vi "RealFlight Controller Layout.vi"(2 "JoyStick Name":string) -> (0 "IDLE up":bool, 1 "Left Lower":bool, 3 "IDLE down":bool, 4 "Down":bool, 5 "Gain":dbl(knob) scale=-1.0..1.0, 6 "Right Stick X":dbl, 7 "Right Stick Y":dbl, 8 "Right":bool, 9 "Left Stick Y":dbl, 10 "Left Stick X":dbl)   [LabVIEW 2012]
uses:
  <vilib>/Rock Robotics/WPI/Joystick/WPI_JoystickGetSetRefNum.vi
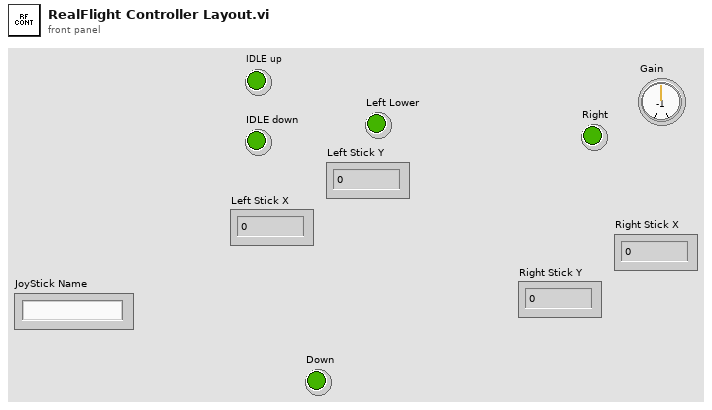
[diagram p1: front panel]
types:
  T1 = typedef "WPI_JoystickDevRef.ctl" = cluster{"Device":T2}
  T2 = typedef "WPI_JoystickDeviceEnum.ctl" = enum16{"USB 1", "USB 2", "USB 3", "USB 4", "Kinect 1", "Kinect 2"}
  T3 = typedef "WPI_JoystickButtonState.ctl" = cluster{"Button 1":bool, "Button 2":bool, "Button 3":bool, "Button 4":bool, "Button 5":bool, "Button 6":bool, "Button 7":bool, "Button 8":bool, "Button 9":bool, "Button 10":bool, "Button 11":bool, "Button 12":bool}
  T4 = cluster{"axis 1 (x)":dbl, "axis 2 (y)":dbl, "axis 3 (throttle)":dbl, "axis 4":dbl, "axis 5":dbl, "axis 6":dbl}
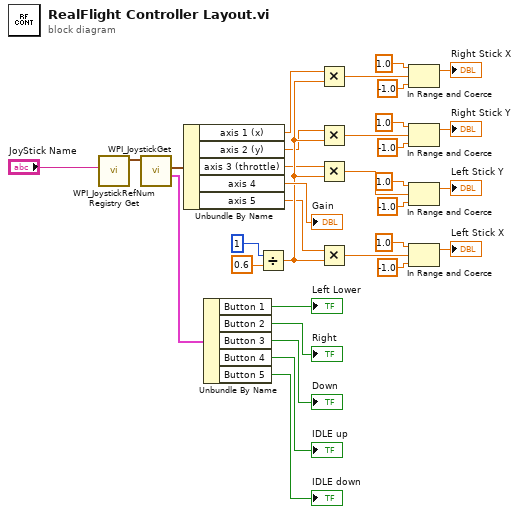
[diagram p0: block diagram]
diagram:
  n1 = call <vilib>:"WPI_JoystickRefNum Registry Get.vi"("refnum name"="JoyStick Name") -> ("JoystickDevRef"=w32:T1)  [unwired: 9 in, 1 out]
  n2 = call <vilib>:"WPI_JoystickGet.vi"("JoystickDevRef"=w32) -> ("Buttons"=w30:T3, "Axes"=w31:T4)  [unwired: 4 in, 1 out]
  n3 = Unbundle By Name(w31) -> ("axis 1 (x)"=w20:dbl, "axis 2 (y)"=w19:dbl, "axis 3 (throttle)"=w18:dbl, "axis 4"=→"Gain":dbl, "axis 5"=w17:dbl)
  n4 = Unbundle By Name(w30) -> ("Button 1"=→"Left Lower":bool, "Button 2"=→"Right":bool, "Button 3"=→"Down":bool, "Button 4"=→"IDLE up":bool, "Button 5"=→"IDLE down":bool)
  n5 = Divide(x=1, y=0.6) -> (x/y=w21:dbl)
  n6 = Multiply(x=w20, y=w21) -> (x*y=w2:dbl)
  n7 = Multiply(x=w19, y=w21) -> (x*y=w4:dbl)
  n8 = Multiply(x=w18, y=w21) -> (x*y=w6:dbl)
  n9 = Multiply(x=w17, y=w21) -> (x*y=w8:dbl)
  n10 = In Range and Coerce(upper limit=1.0, x=w2, lower limit=-1.0 ("upper limit")) -> (coerced(x)=→"Right Stick X":dbl)  [unwired: 1 out]
  n11 = In Range and Coerce(upper limit=1.0, x=w4, lower limit=-1.0 ("upper limit")) -> (coerced(x)=→"Right Stick Y":dbl)  [unwired: 1 out]
  n12 = In Range and Coerce(upper limit=1.0, x=w6, lower limit=-1.0 ("upper limit")) -> (coerced(x)=→"Left Stick Y":dbl)  [unwired: 1 out]
  n13 = In Range and Coerce(upper limit=1.0, x=w8, lower limit=-1.0 ("upper limit")) -> (coerced(x)=→"Left Stick X":dbl)  [unwired: 1 out]
